vi "RH_SCOPE_Close.vi"(8 "error in (no error)":errorcluster, 10 "Reset?":bool, 11 "SCOPE Session In":refnum<k15>) -> (0 "error out":errorcluster)   [LabVIEW 2023, in "ResourceHandling.lvlib"]
doc: "Close Scope session"
uses:
  ResourceHandling.lvlib
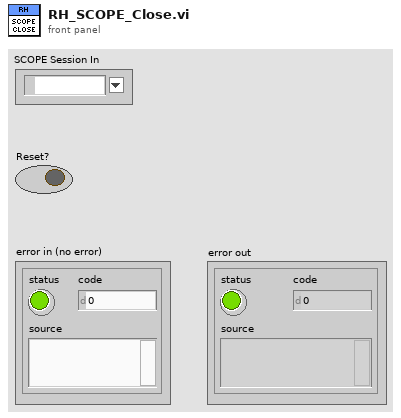
[diagram p1: front panel]
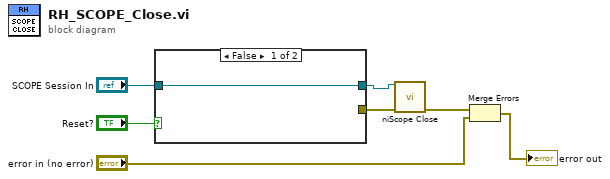
[diagram p0: block diagram]
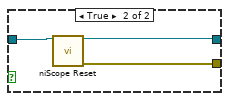
[diagram p2: hidden frame]
diagram:
  n1 = case shown="False" "Reset?" {
    tunnel: [_ w11] -> w6
    tunnel: [w8 w9] -> w2
    tunnel: "SCOPE Session In" -> [w8 w10]
    frame False {
    }
    frame True {
      n2 = call <instrlib>:"niScope Reset.vi"("instrument handle"=w10) -> ("instrument handle out"=w9:refnum<k15>, "error out"=w11:errorcluster)  [unwired: 13 in]
    }
  }
  n3 = call <instrlib>:"niScope Close.vi"("instrument handle"=w2, "error in"=w6) -> ("error out"=w7:errorcluster)  [unwired: 13 in]
  n4 = Merge Errors(w7, "error in (no error)") -> (→"error out":errorcluster)
